vi "SmartSEM Remote API initialize.vi"(8 "error in":errorcluster, 11 "ActiveX Container":refnum<k7>(container)) -> (0 "error out":errorcluster, 3 "reference out":refnum<k7>)   [LabVIEW 2018]
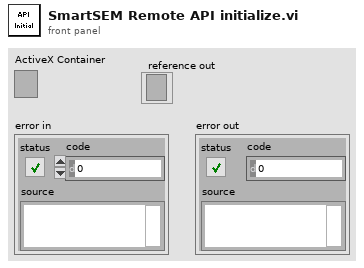
[diagram p1: front panel]
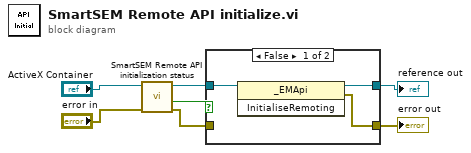
[diagram p0: block diagram]
diagram:
  n1 = call "SmartSEM Remote API initialization status.vi"("error in"="error in", "ActiveX Container"="ActiveX Container") -> ("error out"=w3:errorcluster, "API initialized"=w6:bool, "reference out"=w5:refnum<k7>)  [unwired: 7 in]
  n2 = case shown="False" w6 {
    tunnel: [w9 w12] -> w4
    tunnel: w5 -> [w10 w12]
    tunnel: [w8 w11] -> w2
    tunnel: w3 -> [_ w11]
    frame False {
      n3 = invoke class="_EMApi" method="InitialiseRemoting"(reference=w10) -> (reference out=w9:refnum<k7>, error out=w8:errorcluster)  [unwired: 2 in, 1 out]
    }
    frame True {
    }
  }
  "reference out" <- w4
  "error out" <- w2
